vi "InitializeDAQmxAcquisition.vi.vi"(8 "error in":errorcluster, 10 "cDAQ with TSN AI Channel(s)":tag="Mod1/ai0:3, Mod2/ai0:3", 11 "config in":T1 {"HighPassFilterState"."Filter State" format="%.2f"; "HighPassFilterState"."IIR Filter Cluster"."Forward Coefficients" format="%.2f"; "HighPassFilterState"."IIR Filter Cluster"."Reverse Coefficients" format="%.2f"; "FixedSizeX32"."InputConfig" items=["AC Coupled", "DC Coupled", "IEPE AC Coupled"]}) -> (0 "error out":errorcluster, 3 "config out":T1 {"HighPassFilterState"."Filter State" format="%.2f"; "HighPassFilterState"."IIR Filter Cluster"."Forward Coefficients" format="%.2f"; "HighPassFilterState"."IIR Filter Cluster"."Reverse Coefficients" format="%.2f"; "FixedSizeX32"."InputConfig" items=["AC Coupled", "DC Coupled", "IEPE AC Coupled"]})   [LabVIEW 2017, in "TSNcDAQ_AI.lvlib"]
uses:
  <vilib>/addons/InsightCM/Devices/Shared/Cms/DAQmx/TSNcDAQ_AI.lvlib
  <vilib>/addons/InsightCM/Devices/Shared/Cms/CmsAcquisition/controls/Configuration.ctl
  <vilib>/addons/InsightCM/Devices/Shared/Cms/CmsAcquisition/controls/TachometerConfig.ctl
  <vilib>/addons/InsightCM/Devices/Shared/Cms/CmsAcquisition/controls/FixedSizeArrays.ctl
  <vilib>/LabVIEW Targets/FPGA/cRIO/shared/nicrio_ModuleControls/nicrio_cRIO-9232_ConfigModeRing.ctl
  <vilib>/addons/InsightCM/Devices/Shared/Cms/cRIOWfmAcq/subVIs/RIO Wfm Cust Ctrls/rwfm_SamplingInfo.ctl
  <vilib>/addons/InsightCM/Devices/Shared/Cms/CmsAcquisition/controls/Group.ctl
  <vilib>/addons/InsightCM/Devices/Shared/Cms/CmsAcquisition/controls/Channel.ctl
  <vilib>/addons/InsightCM/Utilities/Analysis/Vibration/controls/HighPassFilterState.ctl
  <vilib>/addons/InsightCM/Devices/Shared/Cms/CmsAcquisition/controls/BurstMode.ctl
  <vilib>/DAQmx/create/channels.llb/DAQmx Create Channel (AI-Voltage-Basic).vi
  <vilib>/DAQmx/configure/timing.llb/DAQmx Timing (Sample Clock).vi
  <vilib>/addons/InsightCM/Devices/Shared/Cms/CmsAcquisition/CmsAcquisition.lvlib
  <vilib>/addons/InsightCM/Devices/Shared/Cms/cRIOWfmAcq/cRIOWfmLib.lvlib
  <vilib>/addons/InsightCM/Utilities/Analysis/Vibration/VibrationAnalysisFunctions.lvlib
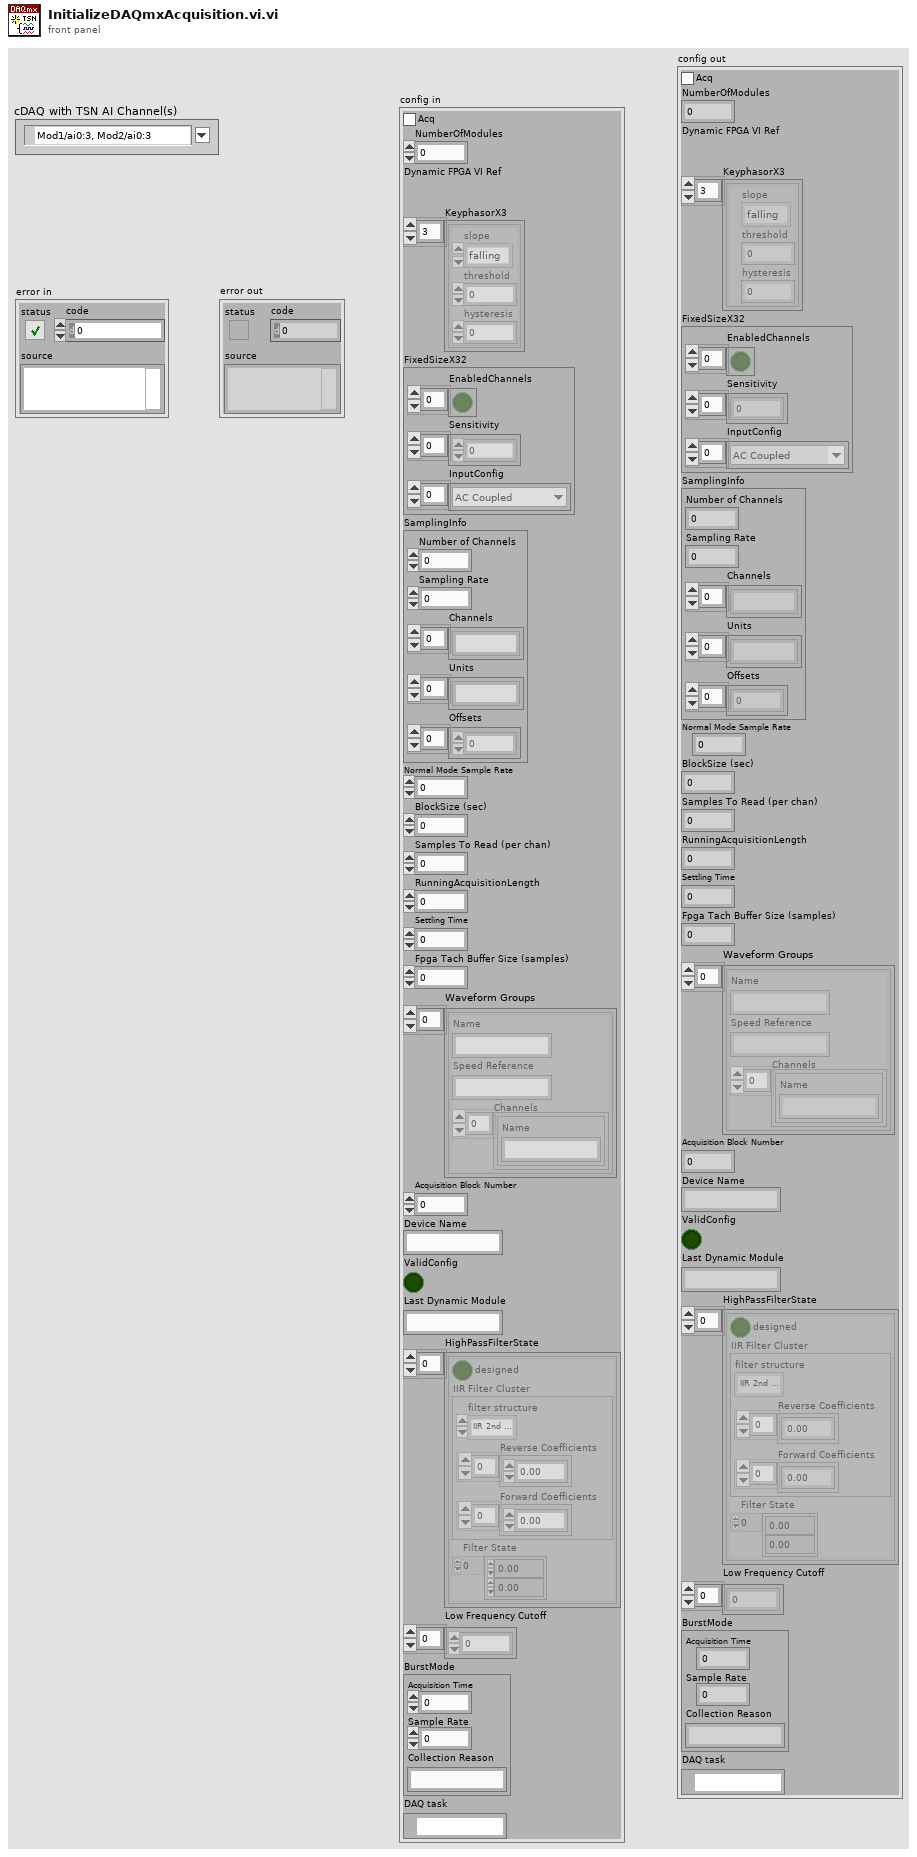
[diagram p1: front panel]
types:
  T1 = typedef "CmsAcquisition.lvlib/Configuration.ctl" = cluster{"Acq":bool, "NumberOfModules":i16, "Dynamic FPGA VI Ref":refnum<k20>, "KeyphasorX3":T2[], "FixedSizeX32":T3, "SamplingInfo":T5, "Normal Mode Sample Rate":dbl, "BlockSize (sec)":dbl, "Samples To Read (per chan)":i32, "RunningAcquisitionLength":dbl, "Settling Time":dbl, "Fpga Tach Buffer Size (samples)":i32, "Waveform Groups":T6[], "Acquisition Block Number":i32, "Device Name":string, "ValidConfig":bool, "Last Dynamic Module":string, "HighPassFilterState":T8[], "Low Frequency Cutoff":dbl[], "BurstMode":T9, "DAQ task":refnum<k21>}
  T2 = typedef "CmsAcquisition.lvlib/TachometerConfig.ctl" = cluster{"slope":enum16{"falling", "rising"}, "threshold":dbl, "hysteresis":dbl}
  T3 = typedef "CmsAcquisition.lvlib/FixedSizeArrays.ctl" = cluster{"EnabledChannels":bool[], "Sensitivity":dbl[], "InputConfig":T4[]}
  T4 = typedef "nicrio_cRIO-9232_ConfigModeRing.ctl" = u8
  T5 = typedef "cRIOWfmLib.lvlib/rwfm_SamplingInfo.ctl" = cluster{"Number of Channels":i32, "Sampling Rate":dbl, "Channels":string[], "Units":string[], "Offsets":sgl[]}
  T6 = typedef "CmsAcquisition.lvlib/Group.ctl" = cluster{"Name":string, "Speed Reference":string, "Channels":T7[]}
  T7 = typedef "CmsAcquisition.lvlib/Channel.ctl" = cluster{"Name":string}
  T8 = typedef "VibrationAnalysisFunctions.lvlib/HighPassFilterState.ctl" = cluster{"designed":bool, "IIR Filter Cluster":cluster{"filter structure":enum32{"IIR 2nd Order", "IIR 4th Order"}, "Reverse Coefficients":dbl[], "Forward Coefficients":dbl[]}, "Filter State":dbl[]}
  T9 = typedef "CmsAcquisition.lvlib/BurstMode.ctl" = cluster{"Acquisition Time":dbl, "Sample Rate":dbl, "Collection Reason":string}
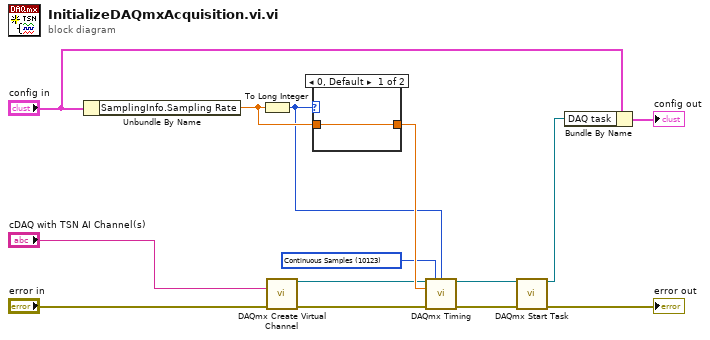
[diagram p0: block diagram]
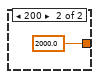
[diagram p2: hidden frame]
diagram:
  w5 = 10123 items=["Finite Samples"=10178, "Continuous Samples"=10123, "Hardware Timed Single Point"=12522] ("Sample Mode")
  n1 = Unbundle By Name("config in") -> ("SamplingInfo.Sampling Rate"=w13:dbl)
  n2 = To Long Integer(number=w13) -> (32bit integer=w1:i32)
  n3 = call-poly <vilib>:"DAQmx Create Virtual Channel.vi"("physical channels"="cDAQ with TSN AI Channel(s)", "error in"="error in") -> ("task out"=w7:refnum<k21>, "error out"=w6:errorcluster)  [unwired: 12 in]
  n4 = case shown="0, Default" w1 {
    tunnel: [w15 2000.0 ("AI Rate (Hz)")] -> w12
    tunnel: w13 -> [w15 _]
    frame 0, Default {
    }
    frame 200 {
    }
  }
  n5 = call-poly <vilib>:"DAQmx Timing.vi"("task/channels in"=w7, "sample mode"=w5, "samples per channel"=w1, "rate"=w12, "error in"=w6) -> ("task out"=w10:refnum<k21>, "error out"=w11:errorcluster)  [unwired: 9 in]
  n6 = call <vilib>:"DAQmx Start Task.vi"("task/channels in"=w10, "error in"=w11) -> ("task out"=w3:refnum<k21>, "error out"=→"error out":errorcluster)  [unwired: 12 in]
  n7 = Bundle By Name(cluster="config in", "DAQ task"=w3) -> (→"config out":T1)
